vi "sandbox.vi"() -> ()   [LabVIEW 2019, in "Inst.KH7008.lvlib" / "Inst.Krohn-Hite-7008.lvclass"]
uses:
  Inst.Krohn-Hite-7008.lvclass
  KH7008/KH7008.lvlib
  <userlib>/LevyLab/LV-Data/LV-Data.PG/LV-Data.PGSQL.lvclass
  KH7008/typedefs/Filter--Enum.ctl
  KH7008/typedefs/couple--Enum.ctl
  KH7008/typedefs/shunt--enum.ctl
  KH7008/typedefs/Input--Enum.ctl
  KH7008/typedefs/gain--enum.ctl
  KH7008/typedefs/channel--numeric.ctl
  KH7008/typedefs/channelProperties--Cluster.ctl
  KH7008/typedefs/allChannelProperties--Array.ctl
  Typedefs/setAllChannelsRequest--Cluster.ctl
  e1ea448e-ba26-459c-8e44-e24a11f284ab.vi
  <vilib>/JDP Science/JSONtext/JSONtext.lvlib
panel:
  in  "Cluster":variant
  out "VCluster out":variant
  out "allChannelProperties":T1 {"channel" min=1 max=8 step=1}
  out "error out":errorcluster
  in  "Channel Parameters out":T1 {"channel" min=1 max=8 step=1}
  in  "stop":bool
  in  "VISA resource name":refnum<visa-resource-name>
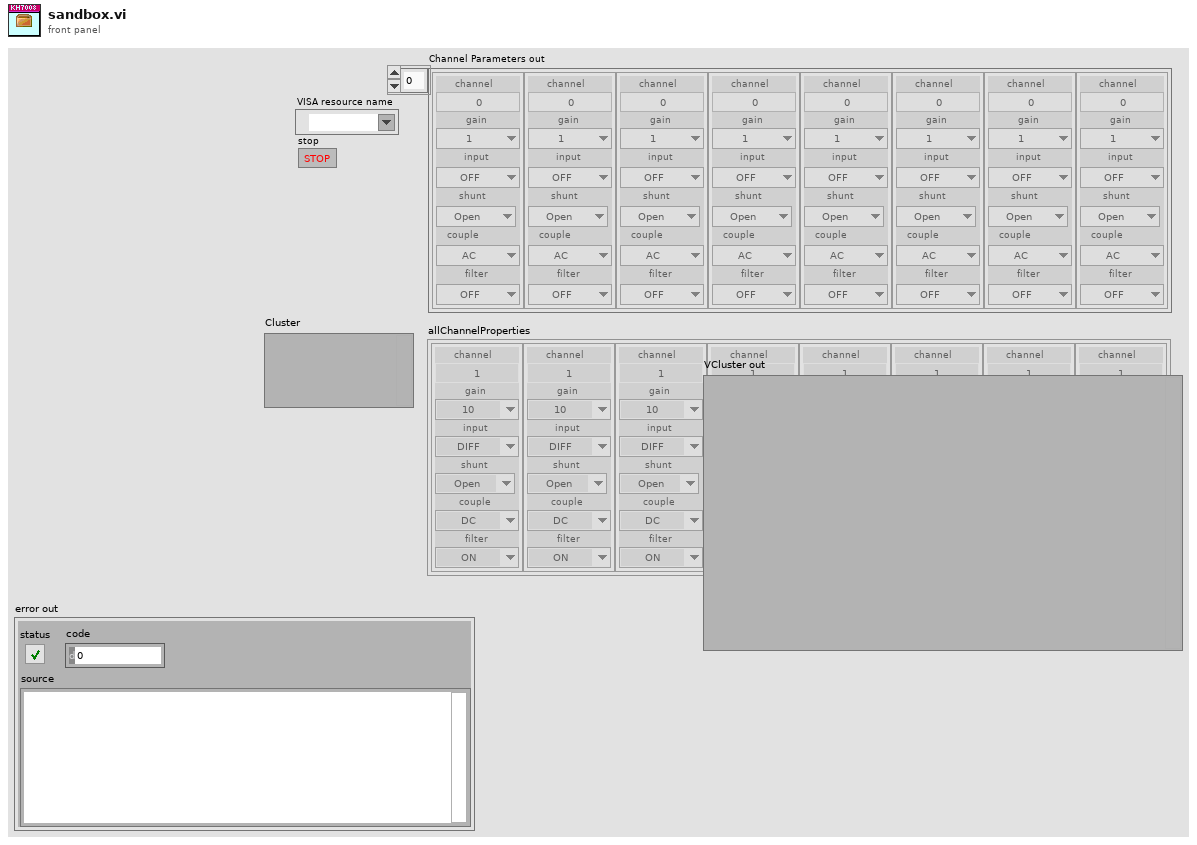
[diagram p1: front panel]
types:
  T1 = typedef "KH7008.lvlib/allChannelProperties--Array.ctl" = T2[]
  T2 = typedef "KH7008.lvlib/channelProperties--Cluster.ctl" = cluster{"channel":T3, "gain":T4, "input":T5, "shunt":T6, "couple":T7, "filter":T8}
  T3 = typedef "KH7008.lvlib/channel--numeric.ctl" = u16
  T4 = typedef "KH7008.lvlib/gain--enum.ctl" = enum16{"1", "10", "100", "1000"}
  T5 = typedef "KH7008.lvlib/input--enum.ctl" = enum16{"OFF", "SE+", "SE-", "DIFF"}
  T6 = typedef "KH7008.lvlib/shunt--enum.ctl" = enum16{"Open", "50", "500", "5k", "50k", "10M"}
  T7 = typedef "KH7008.lvlib/couple--enum.ctl" = enum16{"AC", "DC"}
  T8 = typedef "KH7008.lvlib/filter--enum.ctl" = enum16{"OFF", "ON"}
  T9 = typedef "Inst.KH7008.lvlib/Inst.Krohn-Hite-7008.lvclass/setAllChannelsRequest--Cluster.ctl" = cluster{"allChannelProperties":T1}
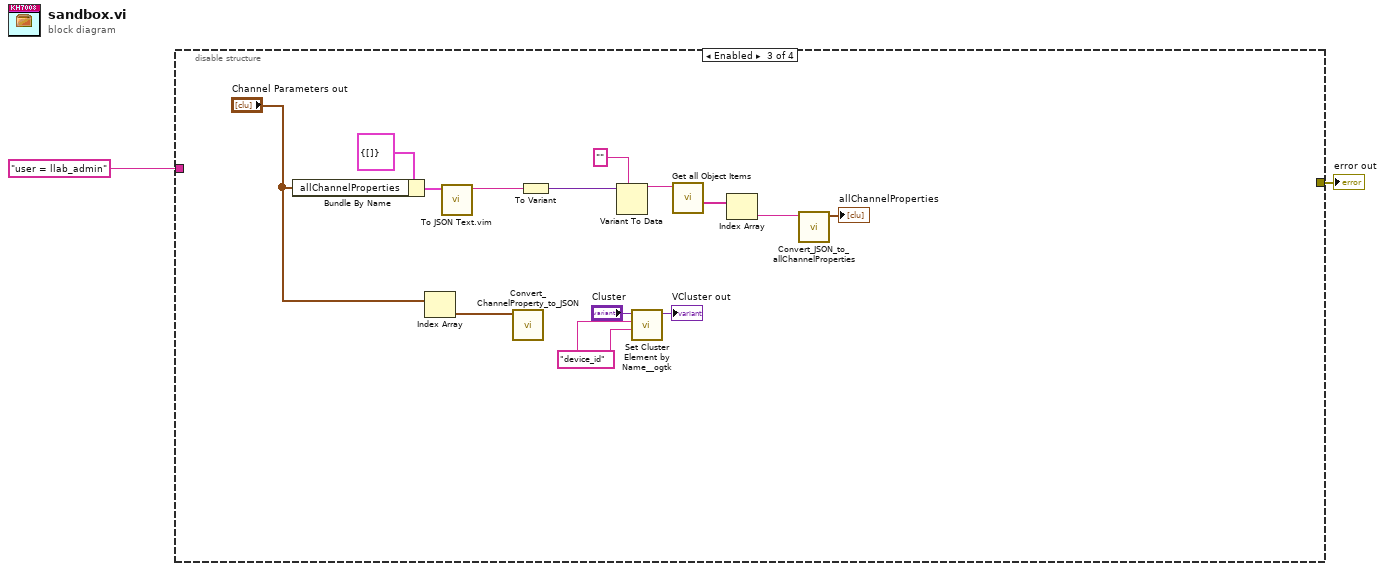
[diagram p0: block diagram]
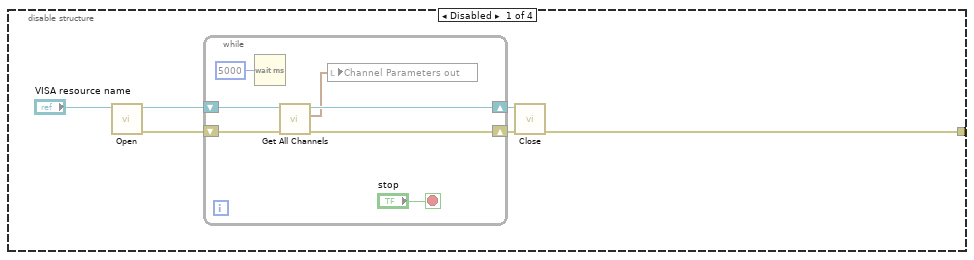
[diagram p2: hidden frame]
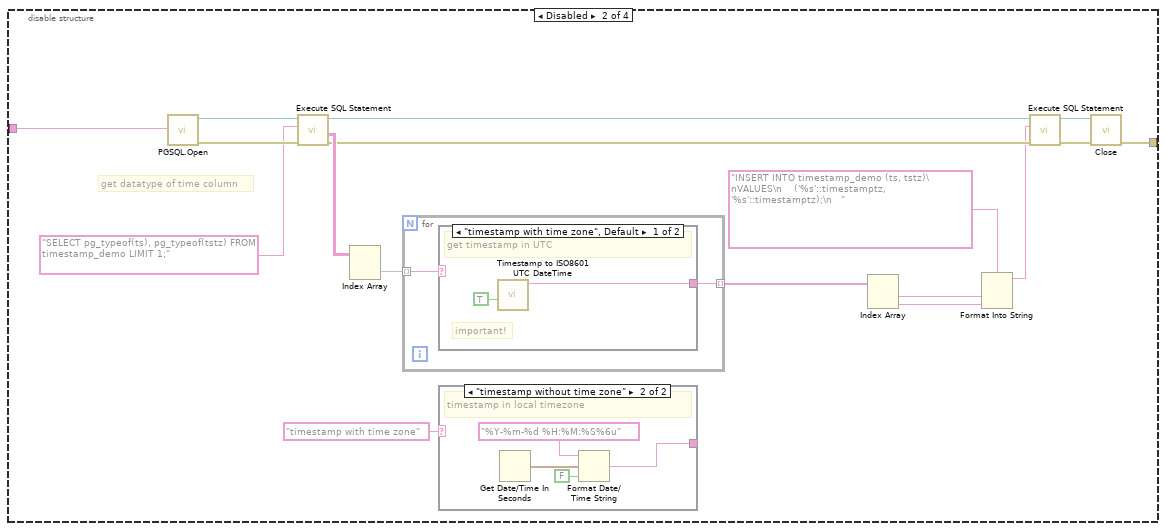
[diagram p3: hidden frame]
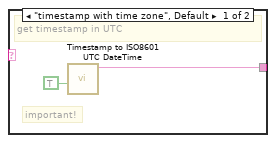
[diagram p4: hidden frame]
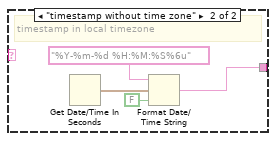
[diagram p5: hidden frame]
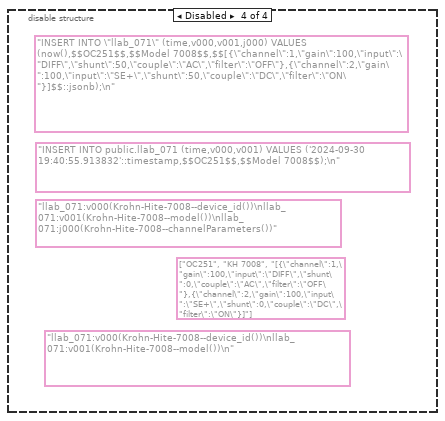
[diagram p6: hidden frame]
diagram:
  n1 = disable-structure shown="Enabled" {
    disable-tunnel: [w3 w30 _ _] -> w2
    disable-tunnel: "user = llab_admin" ("Connection String") -> [_ w19 _ _]
    frame Disabled {
      n2 = call "Open.vi"("VISA resource name"="VISA resource name") -> ("error out"=w6:errorcluster, "VISA resource"=w7:refnum<visa-resource-name>)  [unwired: 9 in]
      n3 = while {
        shift-right: [w13] -> w5
        shift-left: w7 -> [w15]
        shift-right: [w12] -> w4
        shift-left: w6 -> [w14]
        stop <- "stop" stop-if-true
        n4 = Wait (ms)(milliseconds to wait=u32 5000) -> ()  [unwired: 1 out]
        n5 = call "Get All Channels.vi"("error in (no error)"=w14, "VISA Refnum in"=w15) -> ("error out"=w12:errorcluster, "allChannelProperties"=w9:T1, "VISA Refnum out"=w13:refnum<visa-resource-name>)  [unwired: 7 in]
        n6 = local write "Channel Parameters out"(w9) -> ()
      }
      n7 = call "Close.vi"("error in (no error)"=w4, "VISA resource name"=w5) -> ("error out"=w3:errorcluster)  [unwired: 9 in]
    }
    frame Disabled {
      # "get datatype of time column"
      n8 = call <userlib>:"PGSQL.Open.vi"("Connection String"=w19) -> ("error out"=w31:errorcluster, "Data.PG out"=w32:refnum<class "LV-Data.PGSQL.lvclass">)  [unwired: 9 in]
      n9 = call <userlib>:"Execute SQL Statement.vi"("error in (no error)"=w31, "SQL string"="SELECT pg_typeof(ts), pg_typeof(tstz) FROM timestamp_demo LIMIT 1;", "Data.PGQL in"=w32) -> ("error out"=w25:errorcluster, "Result"=w28:string[][], "Data.PGSQL out"=w26:refnum<class "LV-Data.PGSQL.lvclass">)  [unwired: 6 in]
      n10 = Index Array(array=w28) -> (element=w27:string[])  [unwired: 2 in]
      n11 = for {
        tunnel: w27 -> [w40] mode=indexing
        tunnel: [w39] -> w24 mode=indexing
        n12 = case shown="\"timestamp with time zone\", Default" w40 {
          tunnel: [w41 w43] -> w39
          frame "timestamp with time zone", Default {
            # "important!"
            # "get timestamp in UTC"
            n13 = call <vilib>:"Timestamp to ISO8601 UTC DateTime.vi"("UTC? (F)"=TRUE) -> ("ISO8601 String"=w41:string)  [unwired: 10 in]
          }
          frame "timestamp without time zone" {
            # "timestamp in local timezone"
            n14 = Get Date/Time In Seconds() -> (seconds since 1Jan1904=w46:timestamp)
            n15 = Format Date/Time String(time format string (%c)="%Y-%m-%d %H:%M:%S%6u", seconds (now)=w46, UTC format=FALSE) -> (date/time string=w43:string)
          }
        }
      }
      n16 = case shown="\"timestamp without time zone\"" "timestamp with time zone" {
        tunnel: [w33 w35] -> _
        frame "timestamp with time zone", Default {
          # "important!"
          # "get timestamp in UTC"
          n17 = call <vilib>:"Timestamp to ISO8601 UTC DateTime.vi"("UTC? (F)"=TRUE) -> ("ISO8601 String"=w33:string)  [unwired: 10 in]
        }
        frame "timestamp without time zone" {
          # "timestamp in local timezone"
          n18 = Get Date/Time In Seconds() -> (seconds since 1Jan1904=w38:timestamp)
          n19 = Format Date/Time String(time format string (%c)="%Y-%m-%d %H:%M:%S%6u", seconds (now)=w38, UTC format=FALSE) -> (date/time string=w35:string)
        }
      }
      n20 = Index Array(array=w24) -> (element #1=w16:string, element #2=w17:string)  [unwired: 2 in]
      n21 = Format Into String(format string="INSERT INTO timestamp_demo (ts, tstz)\nVALUES\n    ('%s'::timestamptz, '%s'::timestamptz);\n   " ("SQL string"), w16, w17) -> (resulting string=w23:string)  [unwired: 2 in, 1 out]
      n22 = call <userlib>:"Execute SQL Statement.vi"("error in (no error)"=w25, "SQL string"=w23, "Data.PGQL in"=w26) -> ("error out"=w21:errorcluster, "Data.PGSQL out"=w22:refnum<class "LV-Data.PGSQL.lvclass">)  [unwired: 6 in, 1 out]
      n23 = call-dynamic "Close.vi"("error in (no error)"=w21, "Data.PG in"=w22) -> ("error out"=w30:errorcluster)  [unwired: 8 in, 1 out]
    }
    frame Enabled {
      w49 = "device_id" ("Element Name (\"\": New Element Data Name)")
      n24 = Bundle By Name(cluster=T9 {"allChannelProperties"=[]} ("setAllChannelRequest"), "allChannelProperties"="Channel Parameters out") -> (w59:T9)
      n25 = Index Array(array="Channel Parameters out") -> (element=w50:T2)  [unwired: 1 in]
      n26 = call "To JSON Text.vim"("Anything"=w59) -> ("<JSON>"=w54:string)  [unwired: 9 in, 1 out]
      n27 = call "Convert_ChannelProperty_to_JSON.vi"("channelProperties"=w50) -> ()  [unwired: 9 in, 2 out]
      n28 = To Variant(anything=w54) -> (Variant=w53:variant)
      n29 = Variant To Data(type="", Variant=w53) -> (data=w56:string)  [unwired: 1 in, 1 out]
      n30 = call <userlib>:"Set Cluster Element by Name__ogtk.vi"("Element Name (\"\": New Element Data Name)"=w49, "New Element Value"=w49, "Cluster"="Cluster") -> ("VCluster out"=→"VCluster out":variant)  [unwired: 6 in, 2 out]
      n31 = call <vilib>:"Get all Object Items.vi"("JSON"=w56) -> ("<JSON>"=w58:string[])  [unwired: 7 in, 3 out]
      n32 = Index Array(array=w58) -> (element=w57:string)  [unwired: 1 in]
      n33 = call "Convert_JSON_to_allChannelProperties.vi"("<JSON>"=w57) -> ("allChannelProperties"=→"allChannelProperties":T1)  [unwired: 9 in, 1 out]
    }
    frame Disabled {
      (unwired) string[] ["OC251", "KH 7008", "[{\"channel\":1,\"gain\":100,\"input\":\"DIFF\",\"shunt\":0,\"couple\":\"AC\",\"filter\":\"OFF\"},{\"channel\":2,\"gain\":100,\"input\":\"SE+\",\"shunt\":0,\"couple\":\"DC\",\"filter\":\"ON\"}]"] ("SQL string")
      (unwired) "llab_071:v000(Krohn-Hite-7008--device_id())\nllab_071:v001(Krohn-Hite-7008--model())\n" ("SQL string")
      (unwired) "llab_071:v000(Krohn-Hite-7008--device_id())\nllab_071:v001(Krohn-Hite-7008--model())\nllab_071:j000(Krohn-Hite-7008--channelParameters())" ("SQL string")
      (unwired) "INSERT INTO public.llab_071 (time,v000,v001) VALUES ('2024-09-30 19:40:55.913832'::timestamp,$$OC251$$,$$Model 7008$$);\n" ("SQL string")
      (unwired) "INSERT INTO \"llab_071\" (time,v000,v001,j000) VALUES (now(),$$OC251$$,$$Model 7008$$,$$[{\"channel\":1,\"gain\":100,\"input\":\"DIFF\",\"shunt\":50,\"couple\":\"AC\",\"filter\":\"OFF\"},{\"channel\":2,\"gain\":100,\"input\":\"SE+\",\"shunt\":50,\"couple\":\"DC\",\"filter\":\"ON\"}]$$::jsonb);\n" ("SQL string")
    }
  }
  "error out" <- w2
